vi "update_card_FB.vi"(8 "error in (no error)":errorcluster, 10 "Card":bool, 11 "User_Console_States in":refnum<class "User_Console_States.lvclass">) -> (0 "error out":errorcluster, 3 "User_Console_States out":refnum<class "User_Console_States.lvclass">)   [LabVIEW 2025, in "User_Console-ATM.lvlib" / "User_Console_States.lvclass"]
uses:
  User_Console_States.lvclass
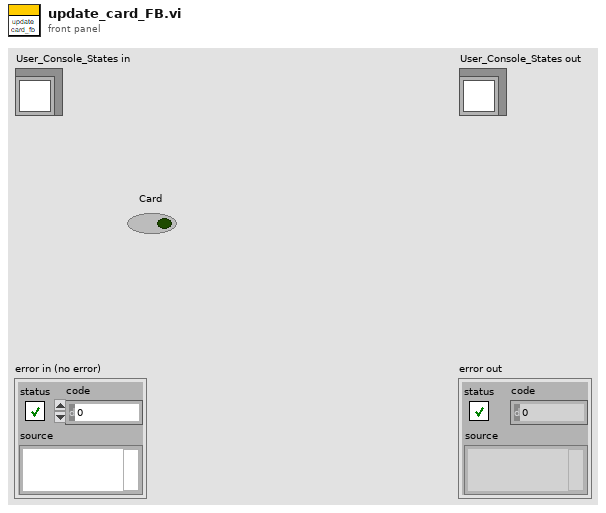
[diagram p1: front panel]
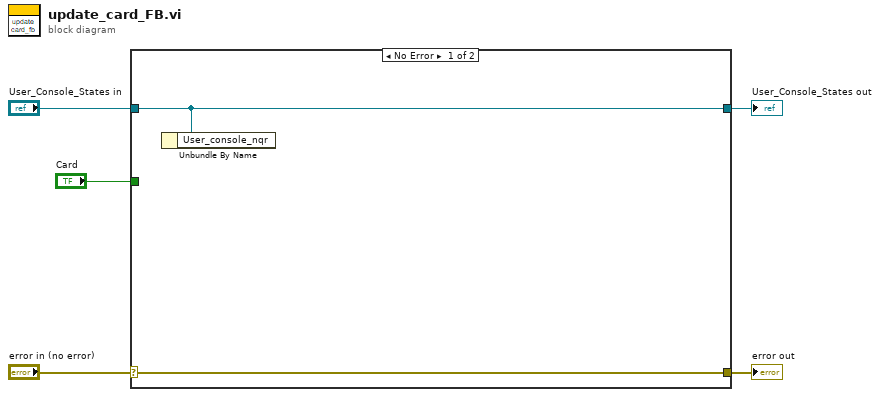
[diagram p0: block diagram]
diagram:
  n1 = case shown="No Error" "error in (no error)" {
    selector: "error in (no error)" -> [w7 w9]
    tunnel: [w7 w9] -> w4
    tunnel: [w6 w8] -> w2
    tunnel: "User_Console_States in" -> [w6 w8]
    tunnel: "Card" -> [_ _]
    frame No Error {
      n2 = Unbundle By Name(w6) -> ()  [unwired: 1 out]
    }
    frame Error {
    }
  }
  "error out" <- w4
  "User_Console_States out" <- w2
